vi "oa_CIC Interpolation with IC.vi"(6 "initial state":cluster{"initial state":dbl[]}[](array[cluster]) {"initial state" format="%.2f"}, 8 "error in (no error)":errorcluster, 10 "CIC filter settings":T1(array[cluster]), 11 "X":dbl[](array[numeric]) format="%.2f") -> (0 "error out":errorcluster, 3 "Y":dbl[](array[numeric]) format="%.2f", 4 "final state":cluster{"final state":dbl[]}[](array[cluster]) {"final state" format="%.2f"})   [LabVIEW 2017, in "SoundVib_Resampling.lvlib"]
uses:
  <vilib>/addons/Sound and Vibration/Order Analysis/Resample Order Tracking/SoundVib_Resampling.lvlib
  <resource>/sndvib.dll
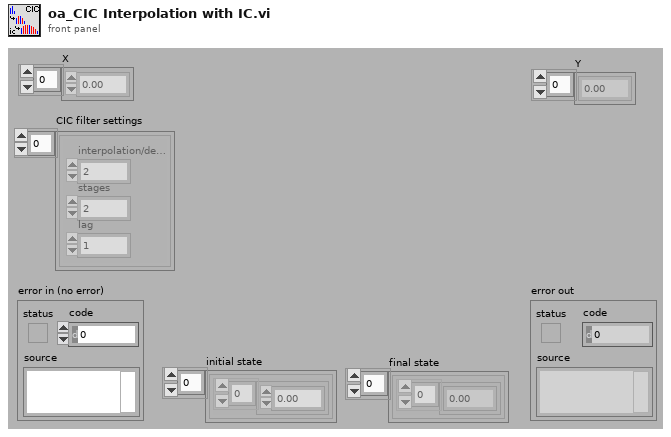
[diagram p1: front panel]
types:
  T1 = cluster{"interpolation/decimation factor":i32, "stages":i32, "lag":i32}[]
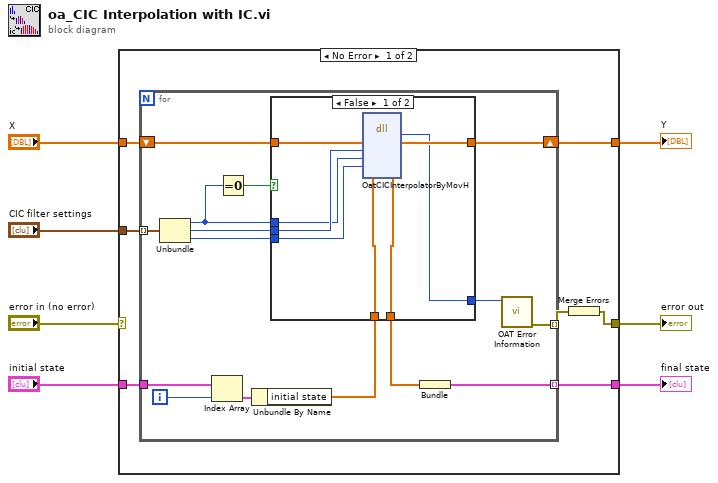
[diagram p0: block diagram]
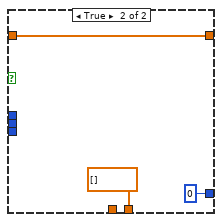
[diagram p2: hidden frame]
diagram:
  n1 = case shown="No Error" "error in (no error)" {
    selector: "error in (no error)" -> [_ w42]
    tunnel: "CIC filter settings" -> [w14 _]
    tunnel: "X" -> [w13 w43]
    tunnel: [w12 w43] -> w5
    tunnel: "initial state" -> [w11 w41]
    tunnel: [w10 w41] -> w3
    tunnel: [w8 w42] -> w2
    frame No Error {
      n2 = for {
        tunnel: w14 -> [w29] mode=indexing
        shift-right: [w26] -> w12
        shift-left: w13 -> [w27]
        tunnel: w11 -> [w25]
        tunnel: [w17] -> w10 mode=indexing
        tunnel: [w15] -> w9 mode=indexing
        i -> [w24]
        n3 = Unbundle(w29) -> ("interpolation/decimation factor"=w20:i32, "stages"=w22:i32, "lag"=w21:i32)
        n4 = Index Array(array=w25, index=w24) -> (element=w23:cluster{"initial state":dbl[]})
        n5 = Equal To 0?(x=w20) -> (x = 0?=w28:bool)
        n6 = Unbundle By Name(w23) -> ("initial state"=w19:dbl[])
        n7 = case shown="False" w28 {
          tunnel: w27 -> [w37 w40]
          tunnel: [w31 w40] -> w26
          tunnel: w22 -> [w36 _]
          tunnel: w21 -> [w35 _]
          tunnel: w20 -> [w34 _]
          tunnel: w19 -> [w33 _]
          tunnel: [w32 dbl[] [] ("initH")] -> w18
          tunnel: [w30 0] -> w16
          frame False {
            n8 = dll-call lib="C:/Program Files (x86)/National Instruments/LabVIEW 2017/resource/sndvib.*" fn="OatCICInterpolatorByMovH"("xH"=w37, "stage"=w36, "dec_factor"=w34, "lag"=w35, "initH"=w33) -> ("return type"=w30:i32, "xH"=w31:dbl[], "initH"=w32:dbl[])  [unwired: 6 in, 2 out]
          }
          frame True {
          }
        }
        n9 = Bundle("initH"=w18) -> (w17:cluster{"initH":dbl[]})  [unwired: 1 in]
        n10 = call <vilib>:"OAT Error Information.vi"("error code"=w16) -> ("error out"=w15:errorcluster)  [unwired: 6 in]
      }
      n11 = Merge Errors(w9) -> (w8:errorcluster)
    }
    frame Error {
    }
  }
  "Y" <- w5
  "final state" <- w3
  "error out" <- w2
